vi "Math-Find Runs.vi"(2 "Min Run Length":i32=2, 3 "Array":bool[](array[boolean])) -> (0 "Length":i32[](array[numeric]), 1 "Start":i32[](array[numeric]))   [LabVIEW 2020]
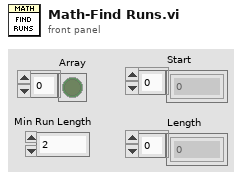
[diagram p1: front panel]
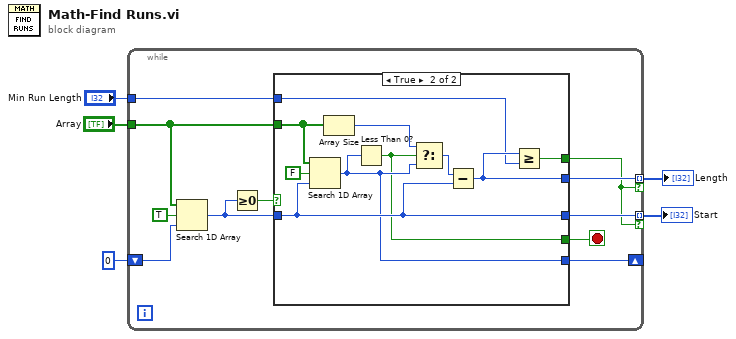
[diagram p0: block diagram]
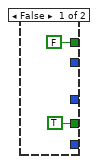
[diagram p2: hidden frame]
diagram:
  n1 = while {
    tunnel: "Array" -> [w15]
    shift-right: [w9] -> _
    shift-left: 0 -> [w14]
    tunnel: [w10] -> w3 mode=indexing if=w6
    tunnel: [w11] -> w2 mode=indexing if=w6
    tunnel: "Min Run Length" -> [w7]
    stop <- w8 stop-if-true
    n2 = Search 1D Array(1D array=w15, element=TRUE, start index (0)=w14) -> (index of element=w13:i32)
    n3 = Greater Or Equal To 0?(x=w13) -> (x >= 0?=w12:bool)
    n4 = case shown="True" w12 {
      tunnel: w15 -> [_ w26]
      tunnel: w13 -> [_ w27]
      tunnel: [_ w27] -> w10
      tunnel: [_ w22] -> w11
      tunnel: [_ w24] -> w9
      tunnel: [TRUE w20] -> w8
      tunnel: w7 -> [_ w21]
      tunnel: [FALSE w19] -> w6
      frame False {
      }
      frame True {
        n5 = Search 1D Array(1D array=w26, element=FALSE, start index (0)=w27) -> (index of element=w24:i32)
        n6 = Array Size(array=w26) -> (size(s)=w23:i32)
        n7 = Less Than 0?(x=w24) -> (x < 0?=w20:bool)
        n8 = Select(t=w23, s=w20, f=w24) -> (s? t:f=w25:i32)
        n9 = Subtract(x=w25, y=w27) -> (x-y=w22:i32)
        n10 = Greater Or Equal?(x=w22, y=w21) -> (x >= y?=w19:bool)
      }
    }
  }
  "Start" <- w3
  "Length" <- w2
